vi "Wait on Stop Sync.vi"(8 "error in (no error)":errorcluster, 10 "Wait for Module to stop?":bool=TRUE, 11 "Module ID":i32) -> (0 "error out":errorcluster)   [LabVIEW 2014, in "GenNet-Client.lvlib"]
doc: "Wait on the rendezvous that synchronizes the request to stop the module and the module stopping.\n\n_____\nBased on Delacor QMH Project Template 3.1.0.34.\n\n<b>Note:</b> This VI was modified by the <b>Validate DQMH Module</b> tool to upgrade it to use an improved stopping mechanism, so that if the user wants to wait until the module stops, the code will only wait for the specific cloneable instance to stop."
uses:
  GenNet-Client.lvlib
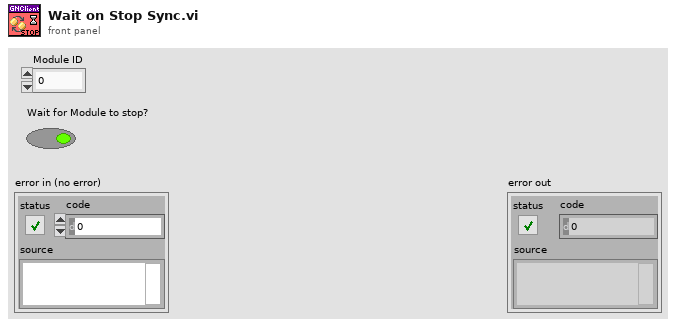
[diagram p1: front panel]
types:
  T1 = typedef "GenNet-Client.lvlib/Broadcast Events--cluster.ctl" = cluster{"Module Did Init":refnum<user-event>, "Status Updated":refnum<user-event>, "Error Reported":refnum<user-event>, "Module Did Stop":refnum<user-event>, "Update Module Execution Status":refnum<user-event>}
  T2 = typedef "Rendezvous RefNum" = refnum<k1>
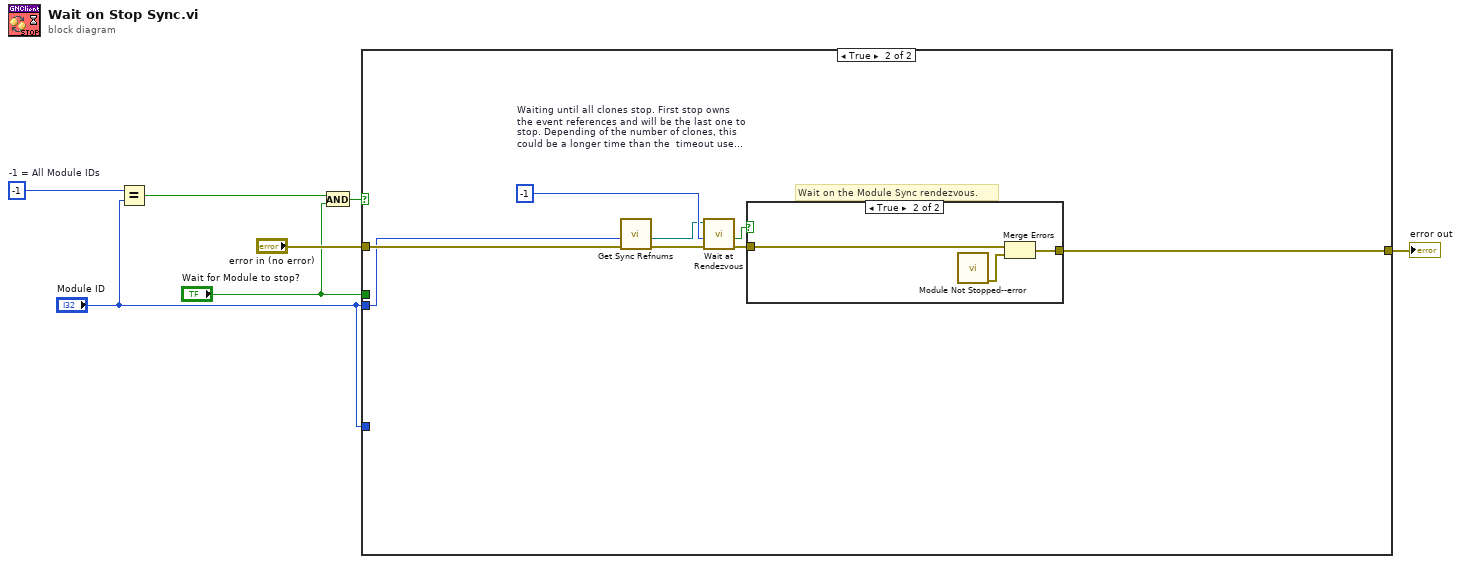
[diagram p0: block diagram]
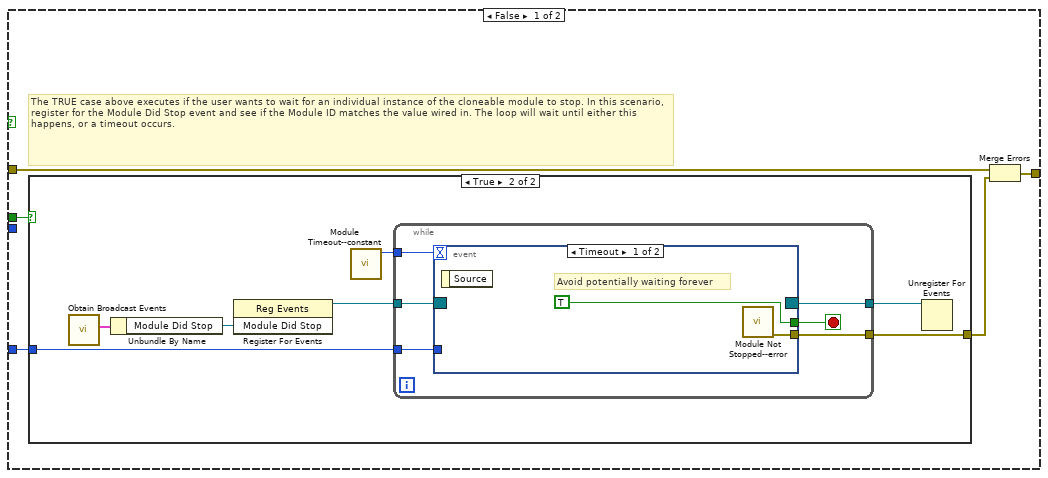
[diagram p2: hidden frame]
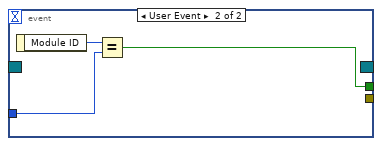
[diagram p4: hidden frame]
diagram:
  w5 = -1  # -1 = All Module IDs
  n1 = Equal?(x=w5, y="Module ID") -> (x = y?=w4:bool)
  n2 = And(x=w4, y="Wait for Module to stop?") -> (x .and. y?=w3:bool)
  n3 = case shown="True" w3 {
    tunnel: "error in (no error)" -> [w12 w38]
    tunnel: [w11 w33] -> w6
    tunnel: "Module ID" -> [_ w32]
    tunnel: "Wait for Module to stop?" -> [w10 _]
    tunnel: "Module ID" -> [w9 _]
    frame False {
      # "The TRUE case above executes if the user wants to wait for an individual instance of the cloneable module to stop. In this scenario, register for the Module Did Stop event and see if the Module ID matches the value wired in. The loop will wait until either this happens, or a timeout occurs."
      n4 = case shown="True" w10 {
        tunnel: w9 -> [_ w17]
        tunnel: [_ w16] -> w8
        frame False {
          # "User does not want to wait for the module to stop."
        }
        frame True {
          n5 = call "Obtain Broadcast Events.vi"() -> ("GenNet-Client Broadcast Events"=w13:T1)  [unwired: 10 in, 1 out]
          n6 = Unbundle By Name(w13) -> ("Module Did Stop"=w19:refnum<user-event>)
          n7 = register-events(w19) -> (reference out=w18:refnum<event-registration>)  [unwired: 2 in, 1 out]
          n8 = call "Module Timeout--constant.vi"() -> ("Module Timeout"=w14:i32)  [unwired: 11 in]
          n9 = while {
            tunnel: w18 -> [w25]
            tunnel: w14 -> [w24]
            tunnel: w17 -> [w22]
            tunnel: [w21] -> w16
            tunnel: [w20] -> w15
            stop <- w23 stop-if-true
            n10 = event shown="[0] Timeout" {
              selector: w25 -> [_ _]
              dyn-events: [_ _] -> w20
              timeout: w24 -> [_ _]
              tunnel: [TRUE w28] -> w23
              tunnel: w22 -> [_ w29]
              tunnel: [w26 _] -> w21
              event Timeout {
                # "Avoid potentially waiting forever"
                n11 = event-data() -> ()  [unwired: 1 in, 1 out]
                n12 = call "Module Not Stopped--error.vi"() -> ("error out"=w26:errorcluster)  [unwired: 11 in]
              }
              event User Event {
                n13 = event-data() -> ("Module ID"=w30:i32)  [unwired: 1 in]
                n14 = Equal?(x=w30, y=w29) -> (x = y?=w28:bool)
              }
            }
          }
          n15 = Unregister For Events(event registration refnum=w15) -> ()  [unwired: 1 in, 1 out]
        }
      }
      n16 = Merge Errors(w12, w8) -> (w11:errorcluster)
    }
    frame True {
      w36 = -1  # Waiting until all clones stop. First stop owns the event references and will be the last one to stop. Depending of the number of clones, this could be a longer time than the  timeout used for the other rendezvous.
      # "Wait on the Module Sync rendezvous."
      n17 = call "Get Sync Refnums.vi"("error in (no error)"=w38, "Module ID"=w32) -> ("error out"=w37:errorcluster, "Stop Sync"=w31:T2)  [unwired: 6 in, 2 out]
      n18 = call <vilib>:"Wait at Rendezvous.vi"("error in (no error)"=w37, "ms timeout (-1)"=w36, "rendezvous"=w31) -> ("error out"=w35:errorcluster, "timed out"=w34:bool)  [unwired: 2 in, 1 out]
      n19 = case shown="True" w34 {
        tunnel: w35 -> [w39 w42]
        tunnel: [w39 w41] -> w33
        frame False {
        }
        frame True {
          n20 = call "Module Not Stopped--error.vi"() -> ("error out"=w40:errorcluster)  [unwired: 11 in]
          n21 = Merge Errors(w42, w40) -> (w41:errorcluster)
        }
      }
    }
  }
  "error out" <- w6
